vi "Practica 12 - FormulaGeneral-SubVI 2.vi"(3 "C":dbl, 4 "B":dbl, 5 "A":dbl) -> (0 "RAIZ 2":dbl, 1 "RAIZ 1":dbl, 2 "TIPO DE RAIZ":string)   [LabVIEW 2020]
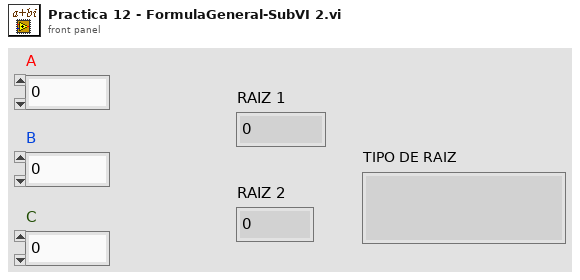
[diagram p1: front panel]
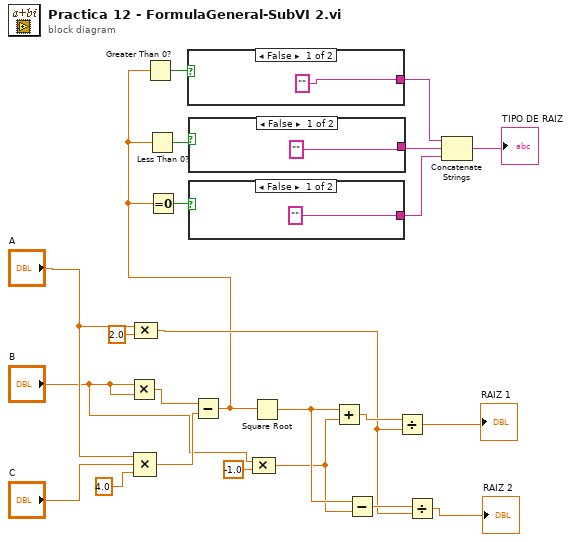
[diagram p0: block diagram]
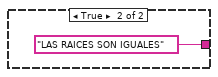
[diagram p2: hidden frame]
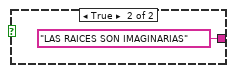
[diagram p3: hidden frame]
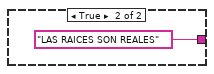
[diagram p4: hidden frame]
diagram:
  n1 = Multiply(x="B", y="B") -> (x*y=w23:dbl)
  n2 = Compound Arithmetic op=MULTIPLY("A", "C", 4.0 ("value")) -> (w20:dbl)
  n3 = Compound Arithmetic op=MULTIPLY("A", 2.0 ("value")) -> (w12:dbl)
  n4 = Subtract(x=w23, y=w20) -> (x-y=w6:dbl)
  n5 = Greater Than 0?(x=w6) -> (x > 0?=w9:bool)
  n6 = Less Than 0?(x=w6) -> (x < 0?=w8:bool)
  n7 = Equal To 0?(x=w6) -> (x = 0?=w7:bool)
  n8 = case shown="False" w9 {
    tunnel: ["" "LAS RAICES SON REALES"] -> w5
    frame False {
    }
    frame True {
    }
  }
  n9 = case shown="False" w8 {
    tunnel: ["" "LAS RAICES SON IMAGINARIAS"] -> w4
    frame False {
    }
    frame True {
    }
  }
  n10 = case shown="False" w7 {
    tunnel: ["" "LAS RAICES SON IGUALES"] -> w3
    frame False {
    }
    frame True {
    }
  }
  n11 = Square Root(x=w6) -> (sqrt(x)=w18:dbl)
  n12 = Compound Arithmetic op=MULTIPLY("B", -1.0 ("value")) -> (w15:dbl)
  n13 = Add(x=w18, y=w15) -> (x+y=w14:dbl)
  n14 = Subtract(x=w18, y=w15) -> (x-y=w13:dbl)
  n15 = Divide(x=w14, y=w12) -> (x/y=→"RAIZ 1":dbl)
  n16 = Divide(x=w13, y=w12) -> (x/y=→"RAIZ 2":dbl)
  n17 = Concatenate Strings(w5, w4, w3) -> (→"TIPO DE RAIZ":string)
